vi "Drivetrain Step Eject Lockout.vi"(9 "Strafe In":dbl, 10 "Steer In":dbl, 11 "Throttle In":dbl) -> (0 "Eject Lockout?":bool, 1 "Strafe Out":dbl, 2 "Steer Out":dbl, 3 "Throttle Out":dbl)   [LabVIEW 2014]
uses:
  Common Code/Auto Roller Commands.ctl
  Common Code/Roller Mode Enum.ctl
  <vilib>/Rock Robotics/WPI/DriverStation/WPI_DriverStationRobotMode2.ctl
  Robot Global Data.vi
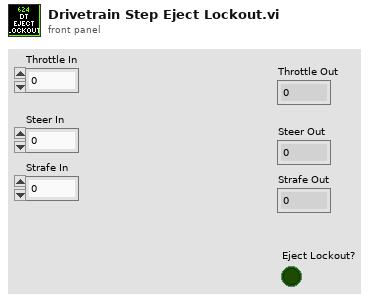
[diagram p1: front panel]
types:
  T1 = typedef "WPI_DriverStationRobotMode2.ctl" = enum16{"Autonomous Disabled", "Autonomous Enabled", "Teleop Disabled", "Teleop Enabled", "Disconnected", "Finish", "Test Disabled", "Test Enabled", "Emergency Stopped"}
  T2 = typedef "Roller Mode Enum.ctl" = enum16{"Manual", "Safe", "Auto"}
  T3 = typedef "Auto Roller Commands.ctl" = enum16{"Grab Tote", "Idle", "Eject Tote", "Untip Can", "Grab Can"}
  T4 = typedef "Roller Indicators.ctl" = cluster{"Rollers Closed?":bool, "Roller Mode":T2, "Auto Roller State":T3, "Tote Inside?":bool, "Intake State":T5, "Left Ping Dist":sgl, "Right Ping Dist":sgl, "Potentiometer Cluster":T6, "PING Decision":T5, "Zero Complete?":bool, "Left Arm Closed?":bool, "Portrait?":bool, "Right Arm Closed?":bool, "Left Out":sgl, "Right Out":sgl, "Left Current":sgl, "Right Current":sgl, "Tote Load Complete?":bool, "Untip Complete?":bool}
  T5 = typedef "Inner Roller States.ctl" = enum16{"Acquire Tote", "Absorb Tote", "Turn Tote Right", "Turn Tote Left"}
  T6 = typedef "Pot Data.ctl" = cluster{"Left Pot Zero":sgl, "Right Pot Zero":sgl, "Left Potentiometer":sgl, "Right Potentiometer":sgl, "Left Pot Non Zero":sgl, "Right Pot Non Zero":sgl}
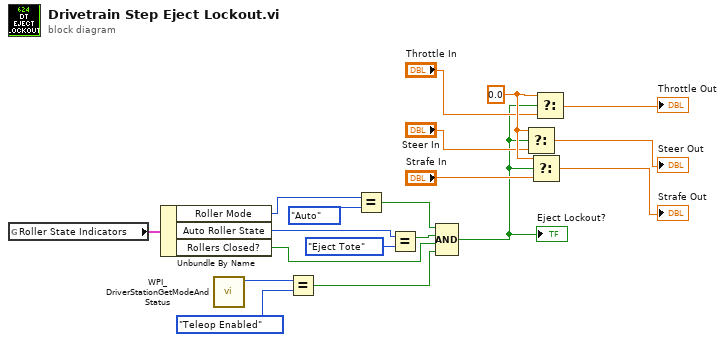
[diagram p0: block diagram]
diagram:
  w19 = 0.0 ("t")
  n1 = global read "Robot Global Data.vi" "Roller State Indicators"() -> (w11:T4)
  n2 = Unbundle By Name(w11) -> ("Roller Mode"=w14:T2, "Auto Roller State"=w12:T3, "Rollers Closed?"=w18:bool)
  n3 = call <vilib>:"WPI_DriverStationGetModeAndStatus.vi"() -> ("Robot Mode"=w3:T1)  [unwired: 10 in, 1 out]
  n4 = Equal?(x=w3, y=WPI_DriverStationRobotMode2."Teleop Enabled") -> (x = y?=w1:bool)
  n5 = Equal?(x=w14, y=Roller_Mode_Enum."Auto") -> (x = y?=w16:bool)
  n6 = Equal?(x=w12, y=Auto_Roller_Commands."Eject Tote") -> (x = y?=w17:bool)
  n7 = Compound Arithmetic op=AND(w16, w17, w18, w1) -> (w4:bool)
  "Eject Lockout?" <- w4
  n8 = Select(t=w19, s=w4, f="Steer In") -> (s? t:f=→"Steer Out":dbl)
  n9 = Select(t=w19, s=w4, f="Strafe In") -> (s? t:f=→"Strafe Out":dbl)
  n10 = Select(t=w19, s=w4, f="Throttle In") -> (s? t:f=→"Throttle Out":dbl)
